vi "matrici_v0_v37.vi"() -> ()   [LabVIEW 2009]
panel:
  out "Valoarea sekectata":bool=TRUE
  in  "Linia":u8(slide)=1 scale=6.0..0.0
  in  "stop":bool
  in  "Coloana":u8(slide)=1 scale=0.0..4.0
  in  "Array":bool[][](array[boolean])=[[TRUE, FALSE, FALSE, FALSE, TRUE], [FALSE, TRUE, FALSE, FALSE, FALSE], [FALSE, FALSE, TRUE, FALSE, FALSE], [FALSE, TRUE, FALSE, FALSE, FALSE], [TRUE, FALSE, FALSE, TRUE, FALSE], [FALSE, FALSE, TRUE, TRUE, FALSE], [TRUE, FALSE, TRUE, TRUE, FALSE]]
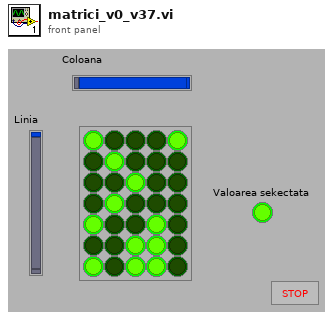
[diagram p1: front panel]
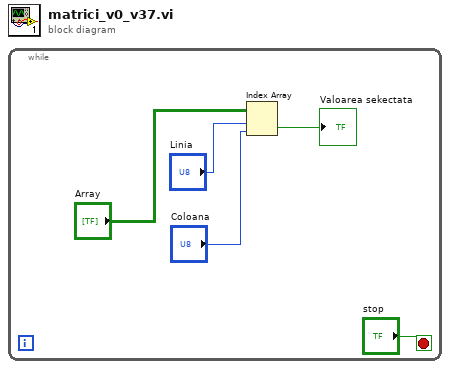
[diagram p0: block diagram]
diagram:
  n1 = while {
    stop <- "stop" stop-if-true
    n2 = Index Array(array="Array", index (row)="Linia", index (col)="Coloana") -> (element=→"Valoarea sekectata":bool)
  }
